vi "testStringToChecksum.vi"() -> ()   [LabVIEW 2016]
uses:
  SerialCommand/CoolerSerialCommand.lvclass
  typedefs/typeOfCommand.ctl
panel:
  in  "String":string=".0101WatchDog"
  out "Checksum":string
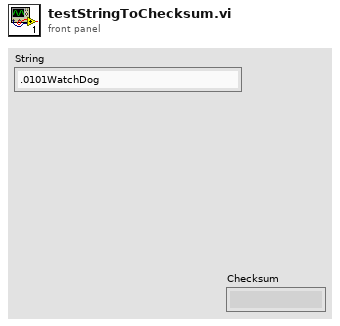
[diagram p1: front panel]
types:
  T1 = typedef "typeOfCommand.ctl" = enum16{"command", "response"}
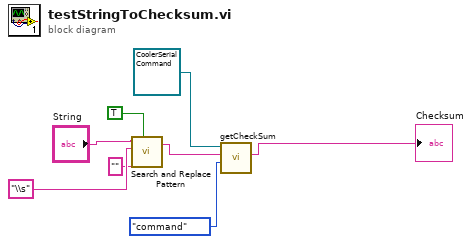
[diagram p0: block diagram]
diagram:
  n1 = call <vilib>:"Search and Replace Pattern.vi"("string"="String", "regular expression (\"\")"="\\s" ("regular expression (\"\")"), "replace string (\"\")"="" ("replace string (\"\")"), "replace all? (F)"=TRUE) -> ("result string"=w5:string)  [unwired: 1 in, 1 out]
  n2 = call "getCheckSum.vi"("messageType"=typeOfCommand."command", "response"=w5, "CoolerSerialCommand in"=refnum<class "CoolerSerialCommand.lvclass"> refnum) -> ("Checksum"=→"Checksum":string)  [unwired: 6 in, 2 out]
